vi "Counter - Read Encoder (Continuous Clock).vi"() -> (0 "error IO":errorcluster)   [LabVIEW 2020]
doc: "This example demonstrates how to use a counter input along with an external clock to continually sample the angular position measured from an encoder.\n\nFor instructions on how to connect your signals to the DAQ device, refer to your device documentation."
uses:
  <vilib>/Utility/error.llb/DialogType.ctl
  <vilib>/DAQmx/read.llb/DAQmx Read (Counter 1D DBL 1Chan NSamp).vi
  <vilib>/DAQmx/create/channels.llb/DAQmx Create Channel (CI-Position-Angular Encoder).vi
  <vilib>/DAQmx/configure/timing.llb/DAQmx Timing (Sample Clock).vi
  <vilib>/DAQmx/miscellaneous.llb/DAQmx Fill In Error Info.vi
  <resource>/objmgr/daqmx.rc
panel:
  in  "Z Index Terminal":tag="PFI9"
  in  "Z Index Enable":bool
  in  "Pulses Per Revolution":u32=24
  in  "B Input Terminal":tag="PFI10"
  in  "A Input Terminal":tag="PFI8"
  in  "Counter":tag="Dev1/ctr0"
  in  "Trigger Type":enum32{"No Trigger", "Digital Arm Start"}(tab)
  in  "Edge":i32(ring)=10280 items=["Rising"=10280, "Falling"=10171]
  in  "Digital Trigger Source":tag
  out "Acquired Data":dbl[](array[numeric])
  in  "Stop":bool
  in  "Samples per Loop":i32=100
  in  "Sample Rate":dbl=1000.0
  in  "Sample Clock Source":tag="PFI0"
  # "Channel Settings"
  # "Acquired Data"
  # "Timing Settings"
  # "Trigger Settings"
  # "To configure and use a trigger or the count reset you must have the necessary tab selected above.  Not all hardware supports the above options--refer to your device documentation for more info."
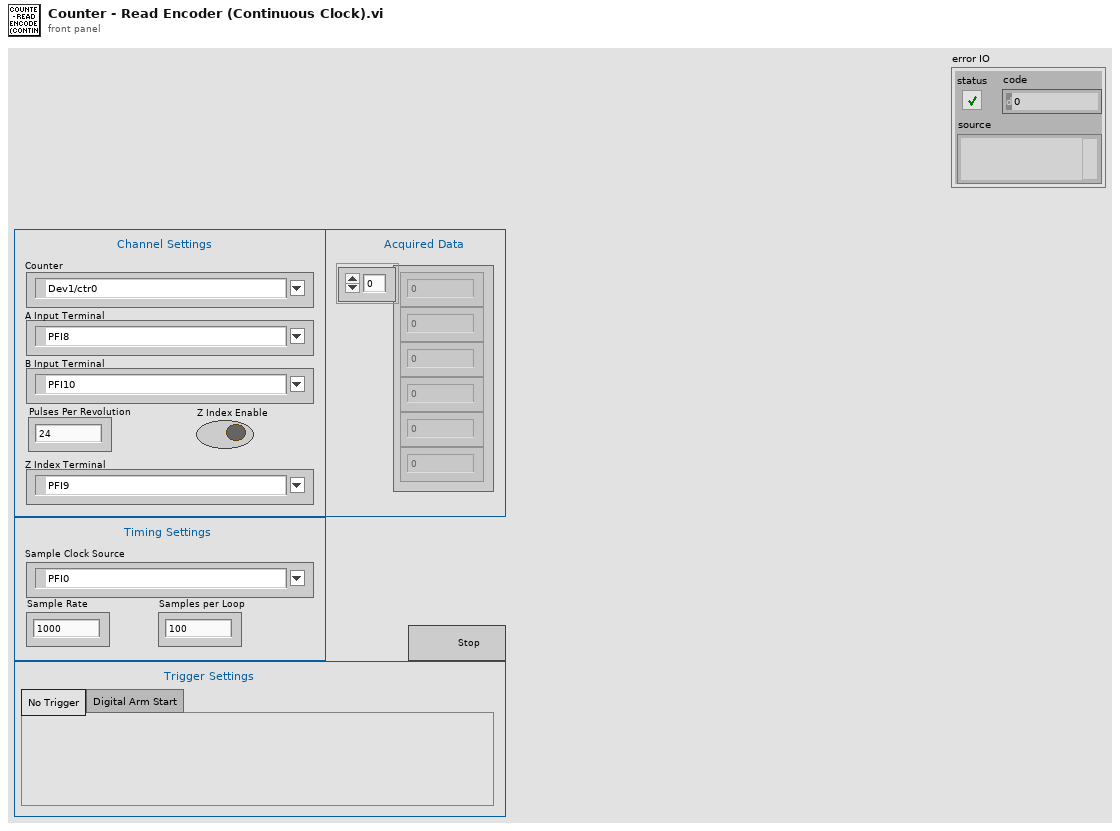
[diagram p1: front panel]
types:
  T1 = typedef "DialogType.ctl" = u16
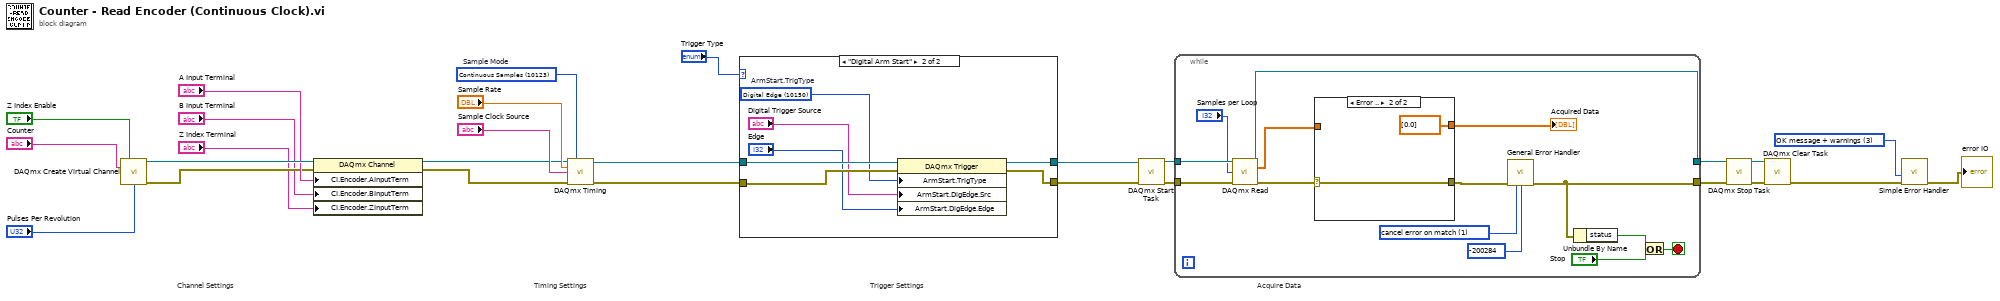
[diagram p0: block diagram]
diagram:
  w3 = T1 3 items=["no dialog", "OK message", "continue or stop message", "OK message + warnings", "continue/stop + warnings"] ("type of dialog (OK msg:1)")
  w27 = 10123 items=["Finite Samples"=10178, "Continuous Samples"=10123, "Hardware Timed Single Point"=12522]  # Sample Mode
  # "Acquire Data"
  # "Trigger Settings"
  # "Timing Settings"
  # "Channel Settings"
  n1 = call-poly <vilib>:"DAQmx Create Virtual Channel.vi"("z index enable"="Z Index Enable", "counter"="Counter", "pulses per revolution"="Pulses Per Revolution") -> ("task out"=w16:refnum<k21>, "error out"=w14:errorcluster)  [unwired: 11 in]
  n2 = property class="DAQmx Channel"(reference=w16, error in=w14, "CI.Encoder.AInputTerm"="A Input Terminal", "CI.Encoder.BInputTerm"="B Input Terminal", "CI.Encoder.ZInputTerm"="Z Index Terminal") -> (reference out=w10:refnum<k21>, error out=w9:errorcluster)
  n3 = call-poly <vilib>:"DAQmx Timing.vi"("task/channels in"=w10, "sample mode"=w27, "rate"="Sample Rate", "source"="Sample Clock Source", "error in"=w9) -> ("task out"=w19:refnum<k21>, "error out"=w18:errorcluster)  [unwired: 9 in]
  n4 = case shown="\"Digital Arm Start\"" "Trigger Type" {
    tunnel: w19 -> [w29 w36]
    tunnel: w18 -> [w28 w33]
    tunnel: [w29 w35] -> w20
    tunnel: [w28 w34] -> w21
    frame "No Trigger", Default {
    }
    frame "Digital Arm Start" {
      w30 = 10150 items=["Digital Edge"=10150, "None"=10230]  # ArmStart.TrigType
      n5 = property class="DAQmx Trigger"(reference=w36, error in=w33, "ArmStart.TrigType"=w30, "ArmStart.DigEdge.Src"="Digital Trigger Source", "ArmStart.DigEdge.Edge"="Edge") -> (reference out=w35:refnum<k21>, error out=w34:errorcluster)
    }
  }
  n6 = call <vilib>:"DAQmx Start Task.vi"("task/channels in"=w20, "error in"=w21) -> ("task out"=w26:refnum<k21>, "error out"=w25:errorcluster)  [unwired: 12 in]
  n7 = while {
    tunnel: w26 -> [w50]
    tunnel: w25 -> [w49]
    tunnel: [w39] -> w6
    tunnel: [w47] -> w7
    stop <- w48 stop-if-true
    w37 = 1 items=["no exception", "cancel error on match", "set error on match"] ("[exception action] (none:0)")
    n8 = call-poly <vilib>:"DAQmx Read.vi"("task/channels in"=w50, "number of samples per channel"="Samples per Loop", "error in"=w49) -> ("task out"=w47:refnum<k21>, "data"=w43:dbl[], "error out"=w41:errorcluster)  [unwired: 10 in]
    n9 = case shown="Error .." w41 {
      selector: w41 -> [w51 w54]
      tunnel: w43 -> [w52 _]
      tunnel: [w52 dbl[] [0.0] ("data")] -> w42
      tunnel: [w51 w54] -> w40
      frame No Error {
      }
      frame Error {
      }
    }
    "Acquired Data" <- w42
    n10 = call <vilib>:"General Error Handler.vi"("error in (no error)"=w40, "[exception action] (none:0)"=w37, "[exception code]"=-200284) -> ("error out"=w39:errorcluster)  [unwired: 8 in, 4 out]
    n11 = Unbundle By Name(w39) -> ("status"=w46:bool)
    n12 = Or(x=w46, y="Stop") -> (x .or. y?=w48:bool)
  }
  n13 = call <vilib>:"DAQmx Stop Task.vi"("task/channels in"=w7, "error in"=w6) -> ("task out"=w4:refnum<k21>, "error out"=w5:errorcluster)  [unwired: 12 in]
  n14 = call <vilib>:"DAQmx Clear Task.vi"("task in"=w4, "error in"=w5) -> ("error out"=w2:errorcluster)  [unwired: 13 in]
  n15 = call <vilib>:"Simple Error Handler.vi"("type of dialog (OK msg:1)"=w3, "error in (no error)"=w2) -> ("error out"=→"error IO":errorcluster)  [unwired: 3 in, 4 out]
